vi "AI Comtinuous Engine Time Testing.vi"   [LabVIEW 2013]
uses:
  Controls/SLL DE Virtual Chart Datalog Driver Options.ctl
  Controls/SLL DE Circular Buffer Pointers List.ctl
  Controls/SLL DE Circular Buffer Options.ctl
types:
  T1 = typedef "SLL DE Virtual Chart Datalog Driver Options.ctl" = enum16{"Initialise", "Write Headings", "Write", "Check File Size", "Read", "Clear"}
  T2 = typedef "SLL DE Circular Buffer Options.ctl" = enum16{"Initialize", "Init Pointer X", "Write", "Read Single Value", "Read Pointer X (Multi Value)", "Clear Data"}
  T3 = typedef "SLL DE Circular Buffer Pointers List.ctl" = enum16{"Graph Pointer", "File Log Pointer", "Pointer 3", "Pointer 4"}
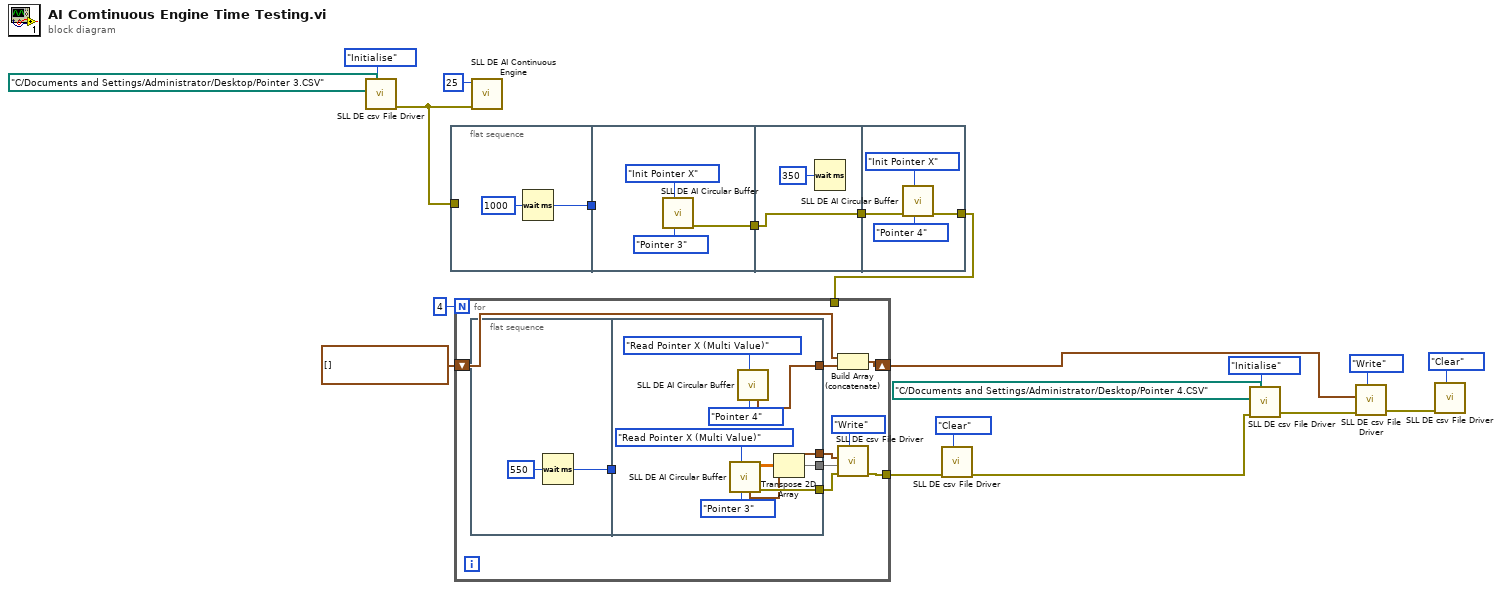
[diagram p0: block diagram]
diagram:
  n1 = call "SLL DE csv File Driver.vi"("Datalog Driver Cases"=SLL_DE_Virtual_Chart_Datalog_Driver_Options."Initialise", "Datalog path (use dialog)"=path "C:/Documents and Settings/Administrator/Desktop/Pointer 3.CSV") -> ("error out"=w17:errorcluster)  [unwired: 5 in, 4 out]
  n2 = flat-sequence {
    tunnel: w17 -> [_]
    tunnel: [w21] -> w16
    tunnel: w16 -> [_]
    tunnel: [w23] -> w12
    tunnel: w12 -> [w27]
    tunnel: [w27] -> w11
    tunnel: w11 -> [w29]
    tunnel: [w28] -> w10
    frame #0 {
      n3 = Wait (ms)(milliseconds to wait=u32 1000) -> (millisecond timer value=w21:u32)
    }
    frame #1 {
      n4 = call "SLL DE AI Circular Buffer.vi"("Pointers"=SLL_DE_Circular_Buffer_Pointers_List."Pointer 3", "Options"=SLL_DE_Circular_Buffer_Options."Init Pointer X") -> ("error Out"=w23:errorcluster)  [unwired: 4 in, 5 out]
    }
    frame #2 {
      n5 = Wait (ms)(milliseconds to wait=u32 350) -> ()  [unwired: 1 out]
    }
    frame #3 {
      n6 = call "SLL DE AI Circular Buffer.vi"("Pointers"=SLL_DE_Circular_Buffer_Pointers_List."Pointer 4", "Options"=SLL_DE_Circular_Buffer_Options."Init Pointer X", "error in (no error)"=w29) -> ("error Out"=w28:errorcluster)  [unwired: 3 in, 5 out]
    }
  }
  n7 = for {
    N: 4 -> [_]
    tunnel: [w37] -> w13
    tunnel: w10 -> [_]
    shift-right: [w33] -> w1
    shift-left: timestamp[] [] -> [w32]
    n8 = flat-sequence {
      tunnel: [w41] -> w40
      tunnel: w40 -> [_]
      tunnel: [w49] -> w38
      tunnel: [w43] -> w36
      tunnel: [w47] -> w35
      tunnel: [w44] -> w34
      frame #0 {
        n9 = Wait (ms)(milliseconds to wait=u32 550) -> (millisecond timer value=w41:u32)
      }
      frame #1 {
        n10 = call "SLL DE AI Circular Buffer.vi"("Pointers"=SLL_DE_Circular_Buffer_Pointers_List."Pointer 3", "Options"=SLL_DE_Circular_Buffer_Options."Read Pointer X (Multi Value)") -> ("error Out"=w49:errorcluster, "Output Data"=w48:sgl[][], "Multi Time Stamp"=w47:timestamp[])  [unwired: 4 in, 3 out]
        n11 = call "SLL DE AI Circular Buffer.vi"("Pointers"=SLL_DE_Circular_Buffer_Pointers_List."Pointer 4", "Options"=SLL_DE_Circular_Buffer_Options."Read Pointer X (Multi Value)") -> ("Multi Time Stamp"=w44:timestamp[])  [unwired: 4 in, 5 out]
        n12 = Transpose 2D Array(2D array=w48) -> (transposed array=w43:sgl[][])
      }
    }
    n13 = Build Array (concatenate)(w32, w34) -> (w33:timestamp[])
    n14 = call "SLL DE csv File Driver.vi"("Datalog Driver Cases"=SLL_DE_Virtual_Chart_Datalog_Driver_Options."Write", "error in(no error)"=w38, "Data In"=w36, "Time Array"=w35) -> ("error out"=w37:errorcluster)  [unwired: 3 in, 4 out]
  }
  n15 = call "SLL DE AI Continuous Engine.vi"("error in (no error)"=w17, "Delay (ms)"=u32 25) -> ()  [unwired: 10 out]
  n16 = call "SLL DE csv File Driver.vi"("Datalog Driver Cases"=SLL_DE_Virtual_Chart_Datalog_Driver_Options."Clear", "error in(no error)"=w13) -> ("error out"=w6:errorcluster)  [unwired: 5 in, 4 out]
  n17 = call "SLL DE csv File Driver.vi"("Datalog Driver Cases"=SLL_DE_Virtual_Chart_Datalog_Driver_Options."Initialise", "error in(no error)"=w6, "Datalog path (use dialog)"=path "C:/Documents and Settings/Administrator/Desktop/Pointer 4.CSV") -> ("error out"=w4:errorcluster)  [unwired: 4 in, 4 out]
  n18 = call "SLL DE csv File Driver.vi"("Datalog Driver Cases"=SLL_DE_Virtual_Chart_Datalog_Driver_Options."Write", "error in(no error)"=w4, "Time Array"=w1) -> ("error out"=w2:errorcluster)  [unwired: 4 in, 4 out]
  n19 = call "SLL DE csv File Driver.vi"("Datalog Driver Cases"=SLL_DE_Virtual_Chart_Datalog_Driver_Options."Clear", "error in(no error)"=w2) -> ()  [unwired: 5 in, 5 out]
